vi "Msg.vi"(7 "Actor in":refnum<class "Actor.lvclass">, 11 "Teardown Error Msg in":refnum<class "Teardown Error Msg.lvclass">) -> (5 "Actor out":refnum<class "Actor.lvclass">)   [LabVIEW 2020, in "jettl.lvlib" / "Teardown Error Msg.lvlib" / "Teardown Error Msg.lvclass"]
uses:
  Teardown Error Msg.lvclass
  Teardown Error/Teardown Error.lvclass
  Actor/Actor/Actor.lvclass
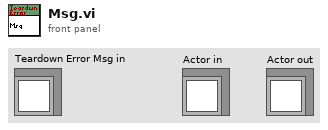
[diagram p1: front panel]
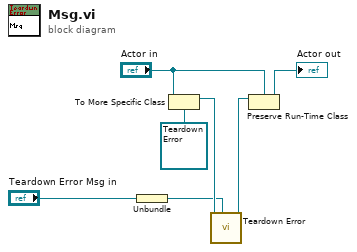
[diagram p0: block diagram]
diagram:
  n1 = Unbundle "Unbundle"("Teardown Error Msg in") -> (w1:refnum<class "Sender.lvclass">)
  n2 = To More Specific Class(target class=refnum<class "Teardown Error.lvclass"> refnum ("Destroy.lvlib:Destroy.lvclass"), reference="Actor in") -> (specific class reference=w3:refnum<class "Teardown Error.lvclass">)  [unwired: 1 in, 1 out]
  n3 = call-dynamic "Teardown Error.vi"("Sender"=w1, "Teardown Error in"=w3) -> ("Teardown Error out"=w2:refnum<class "Teardown Error.lvclass">)  [unwired: 9 in]
  n4 = Preserve Run-Time Class(object in=w2, 2:"Actor in") -> (object out=→"Actor out":refnum<class "Actor.lvclass">)  [unwired: 1 in, 1 out]
